vi "VIListReloadEnumVIs.vi"(8 "error in (no error)":errorcluster, 11 "Application in":refnum<vi>) -> (0 "error out":errorcluster, 1 "Paths":string[](array[string]), 2 "VI Tags":string[](array[string]), 3 "Application out":refnum<vi>)   [LabVIEW 2019, in "VIPropertyPicker.lvlib"]
uses:
  VIPropertyPicker.lvlib
  b5b0ca77-5f3c-4af6-9f2c-4ccc2142e757.vi
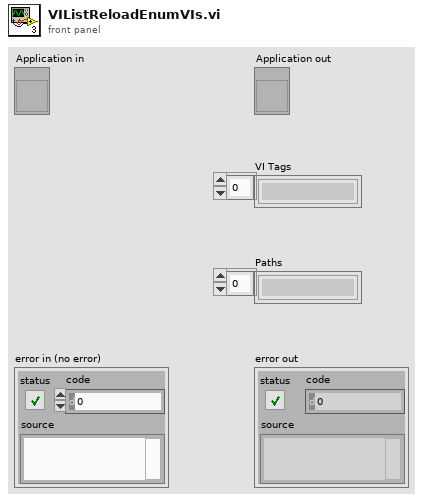
[diagram p1: front panel]
types:
  T1 = enum32{"Bad", "Idle", "Run top level", "Running"}
  T2 = enum32{"Bad", "Idle", "Run top level", "Running"}[]
  T3 = enum32{"Invalid", "Standard", "Closed", "Hidden", "Minimized", "Maximized"}
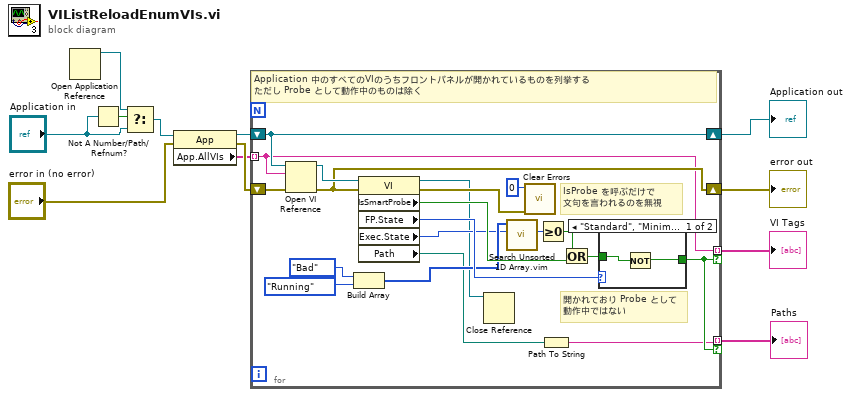
[diagram p0: block diagram]
diagram:
  n1 = Open Application Reference() -> (3:w2:refnum<vi>)  [unwired: 4 in, 1 out]
  n2 = Not A Number/Path/Refnum?(number/path/refnum="Application in") -> (NaN/Path/Refnum?=w5:bool)
  n3 = Select(t=w2, s=w5, f="Application in") -> (s? t:f=w3:refnum<vi>)
  n4 = property class="App"(reference=w3, error in="error in (no error)") -> (reference out=w8:refnum<vi>, error out=w11:errorcluster, "App.AllVIs"=w9:string[])
  n5 = for {
    tunnel: w9 -> [w26] mode=indexing
    shift-right: [w30] -> w12
    shift-left: w11 -> [w31]
    shift-right: [w27] -> w7
    shift-left: w8 -> [w27]
    tunnel: [w26] -> w6 mode=indexing if=w25
    tunnel: [w14] -> w1 mode=indexing if=w25
    # "開かれており Probe として\n動作中ではない"
    # "IsProbe を呼ぶだけで\n文句を言われるのを無視"
    # "Application 中のすべてのVIのうちフロントパネルが開かれているものを列挙する\nただし Probe として動作中のものは除く"
    n6 = Open VI Reference(application reference (local)=w27, vi path=w26, error in (no error)=w31) -> (vi reference=w32:refnum<vi>, error out=w30:errorcluster)  [unwired: 3 in]
    n7 = Build Array(T1."Bad" ("Execution:State"), T1."Running" ("Execution:State")) -> (w20:T2)
    n8 = property class="VI"(reference=w32, error in=w30) -> (reference out=w13:refnum<vi>, error out=w29:errorcluster, "IsSmartProbe"=w24:bool, "FP.State"=w23:T3, "Exec.State"=w19:T1, "Path"=w15:path)
    n9 = Close Reference(reference=w13) -> ()  [unwired: 1 in, 1 out]
    n10 = call "Search Unsorted 1D Array.vim"("element"=w19, "unsorted 1D array"=w20) -> ("index of element"=w18:i32)  [unwired: 9 in]
    n11 = call <vilib>:"Clear Errors.vi"("error in (no error)"=w29, "specific error code to clear (0: all)"=0) -> ()  [unwired: 4 in, 2 out]
    n12 = Greater Or Equal To 0?(x=w18) -> (x >= 0?=w16:bool)
    n13 = Path To String(path=w15) -> (string=w14:string)
    n14 = Or(x=w16, y=w24) -> (x .or. y?=w17:bool)
    n15 = case shown="\"Standard\", \"Minimized\", \"Maximized\"" w23 {
      tunnel: [w34 _] -> w25
      tunnel: w17 -> [w33 _]
      frame "Standard", "Minimized", "Maximized" {
        n16 = Not(x=w33) -> (.not. x?=w34:bool)
      }
      frame Default {
      }
    }
  }
  "VI Tags" <- w6
  "error out" <- w12
  "Application out" <- w7
  "Paths" <- w1
